vi "solar_gbl Launch Splash.vi"(8 "error in (no error)":errorcluster, 11 "SOLAR in":T1) -> (0 "error out":errorcluster, 2 "Splash VI Refnum":refnum<vi>, 3 "SOLAR out":T1)   [LabVIEW 2018]
doc: "This launches the SOLAR splash screen. Change the splash screen image in the solar.ini configuration file."
uses:
  solar_ctl SOLAR Global.ctl
  solar_ctl Target Global.ctl
  voyager/solar_voy_ctl Voyager Refnum.ctl
  qtimer/solar_qtimer_ctl Refnum.ctl
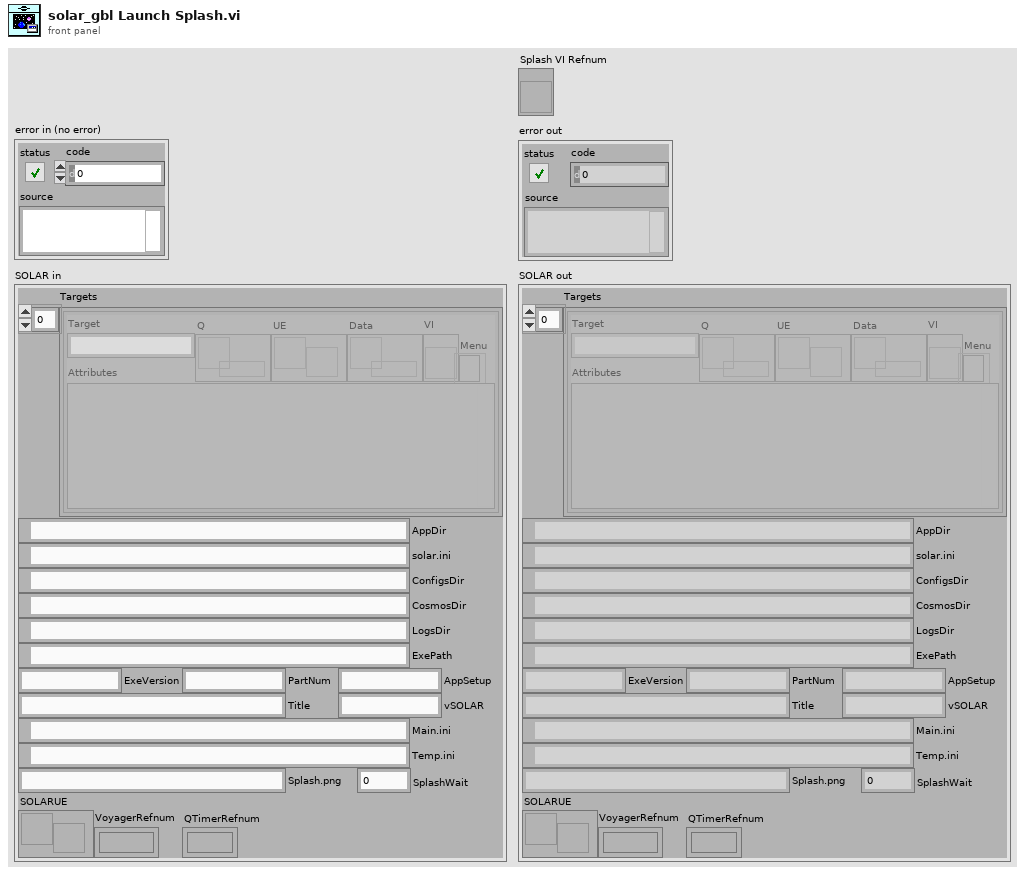
[diagram p1: front panel]
types:
  T1 = typedef "solar_ctl SOLAR Global.ctl" = cluster{"Targets":T2[], "AppDir":path, "solar.ini":path, "ConfigsDir":path, "CosmosDir":path, "LogsDir":path, "ExePath":path, "ExeVersion":string, "PartNum":string, "AppSetup":string, "Title":string, "Main.ini":path, "Temp.ini":path, "vSOLAR":string, "Splash.png":string, "SplashWait":i32, "SOLARUE":refnum<user-event>, "VoyagerRefnum":T3, "QTimerRefnum":T4}
  T2 = typedef "solar_ctl Target Global.ctl" = cluster{"Target":string, "Q":refnum<queue>, "UE":refnum<user-event>, "VI":refnum<vi>, "Menu":refnum<k9>, "Data":refnum<data-value>, "Attributes":variant}
  T3 = typedef "solar_voy_ctl Voyager Refnum.ctl" = refnum<k1>
  T4 = typedef "solar_qtimer_ctl Refnum.ctl" = refnum<k1>
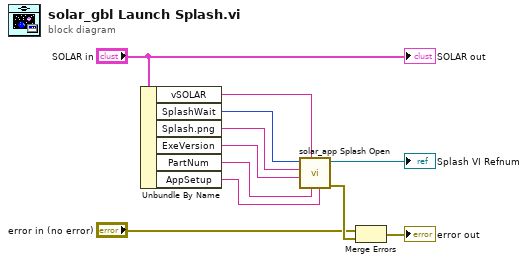
[diagram p0: block diagram]
diagram:
  n1 = Unbundle By Name("SOLAR in") -> ("vSOLAR"=w2:string, "SplashWait"=w7:i32, "Splash.png"=w6:string, "ExeVersion"=w5:string, "PartNum"=w4:string, "AppSetup"=w3:string)
  n2 = call "solar_app Splash Open.vi"("App Setup"=w3, "Part Number"=w4, "SOLAR Version"=w2, "Exe Version"=w5, "Splash Path (\"\")"=w6, "Splash msWait (-1)"=w7) -> ("error out"=w10:errorcluster, "Splash VI Refnum"=→"Splash VI Refnum":refnum<vi>)  [unwired: 4 in]
  n3 = Merge Errors("error in (no error)", w10) -> (→"error out":errorcluster)
  "SOLAR out" <- "SOLAR in"
